vi "Method 1.vi"(8 "error in (no error)":errorcluster, 11 "Child in":refnum<class "Child.lvclass">) -> (0 "error out":errorcluster, 3 "Child out":refnum<class "Child.lvclass">)   [LabVIEW 2021, in "Child.lvclass"]
uses:
  Child.lvclass
  Child.lvclass/Child.ctl
  Interface/Interface.lvclass
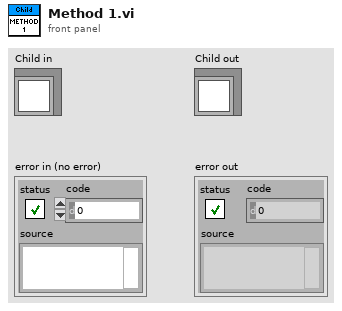
[diagram p1: front panel]
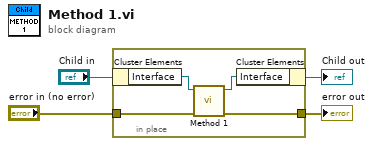
[diagram p0: block diagram]
diagram:
  n1 = in-place {
    in-place-border: [w6] -> w2
    in-place-border: "error in (no error)" -> [w5]
    n2 = in-place-cluster #1("Child in") -> ("Interface"=w8:refnum<class "Interface.lvclass">)
    n3 = call-dynamic "Method 1.vi"("error in (no error)"=w5, "Interface 1 in"=w8) -> ("error out"=w6:errorcluster, "Interface 1 out"=w7:refnum<class "Interface.lvclass">)  [unwired: 8 in]
    n4 = in-place-cluster #1("Interface"=w7) -> (→"Child out":refnum<class "Child.lvclass">)
  }
  "error out" <- w2
